vi "LaunchGenerator.vi"() -> ()   [LabVIEW 2014]
uses:
  <vilib>/ActorFramework/Actor/Actor.lvclass
  Generator/Generator/Generator.lvclass
  Generator/Generator Messages/GetDateTimeString Msg/GetDateTimeString Msg.lvclass
  Generator/Generator Messages/GetRandomNum Msg/GetRandomNum Msg.lvclass
  Generator/Generator Messages/GetRandomString Msg/GetRandomString Msg.lvclass
  <vilib>/ActorFramework/Stop Msg/Stop Msg.lvclass
  Generator/Generator Messages/Write NumRange Msg/Write NumRange Msg.lvclass
  Generator/Generator Messages/Write StringLength Msg/Write StringLength Msg.lvclass
  7fd6c2e3-5a34-4bbf-a67f-205d0afb060b.vi
panel:
  in  "stop":bool
  out "RandomString":string
  out "RandomNum":dbl
  out "DateTimeString":string
  in  "StringLength":i32
  in  "NumRange":dbl
  # "Launch VI"
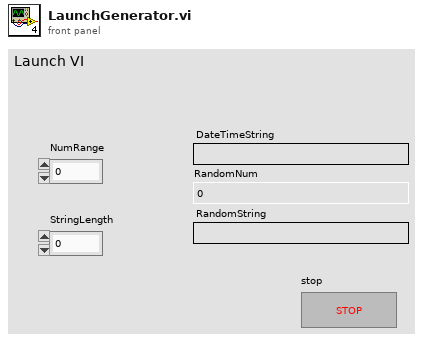
[diagram p1: front panel]
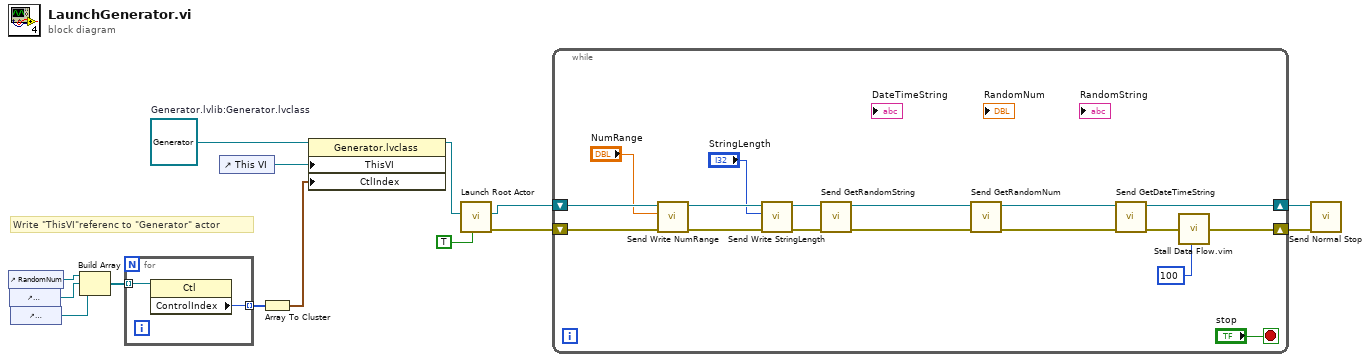
[diagram p0: block diagram]
diagram:
  w14 = refnum<class "Generator.lvclass"> refnum  # Generator.lvlib:Generator.lvclass
  # "Write \"ThisVI\"referenc to \"Generator\" actor"
  n1 = control-ref of="RandomNum"() -> (w2:refnum<vi>)
  n2 = control-ref of="RandomString"() -> (w1:refnum<vi>)
  n3 = control-ref of="DateTimeString"() -> (w6:refnum<vi>)
  n4 = Build Array(w2, w1, w6) -> (w5:refnum<vi>[])
  n5 = for {
    tunnel: w5 -> [w16] mode=indexing
    tunnel: [w15] -> w4 mode=indexing
    n6 = property class="Ctl"(reference=w16) -> ("ControlIndex"=w15:i32)  [unwired: 1 in, 2 out]
  }
  n7 = control-ref of="This VI"() -> (w7:refnum<vi>)
  n8 = Array To Cluster(array=w4) -> (cluster=w3:cluster{"[0]":i32, "[1]":i32, "[2]":i32})
  n9 = property class="Generator.lvclass"(reference=w14, "ThisVI"=w7, "CtlIndex"=w3) -> (reference out=w8:refnum<class "Generator.lvclass">)  [unwired: 1 in, 1 out]
  n10 = call <vilib>:"Launch Root Actor.vi"("Open Actor Core front panel? (F)"=TRUE, "Actor"=w8) -> ("error out"=w13:errorcluster, "Actor's Enqueuer"=w11:refnum<class "Message Enqueuer.lvclass">)  [unwired: 8 in]
  n11 = while {
    shift-right: [w19] -> w9
    shift-left: w13 -> [w33]
    shift-right: [w21] -> w10
    shift-left: w11 -> [w27]
    stop <- "stop" stop-if-true
    n12 = call "Send Write NumRange.vi"("error in (no error)"=w33, "NumRange"="NumRange", "Message Enqueuer"=w27) -> ("error out"=w28:errorcluster, "Message Enqueuer out"=w24:refnum<class "Message Enqueuer.lvclass">)  [unwired: 7 in]
    n13 = call "Send Write StringLength.vi"("error in (no error)"=w28, "StringLength"="StringLength", "Message Enqueuer"=w24) -> ("error out"=w25:errorcluster, "Message Enqueuer out"=w23:refnum<class "Message Enqueuer.lvclass">)  [unwired: 7 in]
    n14 = call "Send GetRandomString.vi"("error in (no error)"=w25, "Message Enqueuer"=w23) -> ("error out"=w31:errorcluster, "Message Enqueuer out"=w32:refnum<class "Message Enqueuer.lvclass">)  [unwired: 8 in]
    n15 = call "Send GetRandomNum.vi"("error in (no error)"=w31, "Message Enqueuer"=w32) -> ("error out"=w29:errorcluster, "Message Enqueuer out"=w30:refnum<class "Message Enqueuer.lvclass">)  [unwired: 8 in]
    n16 = call "Send GetDateTimeString.vi"("error in (no error)"=w29, "Message Enqueuer"=w30) -> ("error out"=w20:errorcluster, "Message Enqueuer out"=w21:refnum<class "Message Enqueuer.lvclass">)  [unwired: 8 in]
    n17 = call "Stall Data Flow.vim"("value in"=w20, "milliseconds to wait"=u32 100) -> ("value out"=w19:errorcluster)  [unwired: 1 out]
  }
  n18 = call <vilib>:"Send Normal Stop.vi"("error in (no error)"=w9, "Message Enqueuer"=w10) -> ()  [unwired: 9 in, 1 out]
